vi "convert to deltaF-F.vi"(8 "error in (no error)":errorcluster, 11 "DAQOrcaFlash in":refnum<class "DAQOrcaFlash.lvclass">) -> (0 "error out":errorcluster, 3 "DAQOrcaFlash out":refnum<class "DAQOrcaFlash.lvclass">)   [LabVIEW 2012, in "DAQOrcaFlash.lvclass"]
uses:
  DAQOrcaFlash.lvclass
  dependencies/LabTIFF/LabTIFF/Opening Purpose.ctl
  DAQOrcaFlash.lvclass/DAQOrcaFlash.ctl
panel:
  out "min value":u32
  out "max value":u32
  out "file progress":dbl(slide) scale=0.0..1.0
  out "folder progress":dbl(slide) scale=0.0..1.0
  in  "cxd folder Path":path
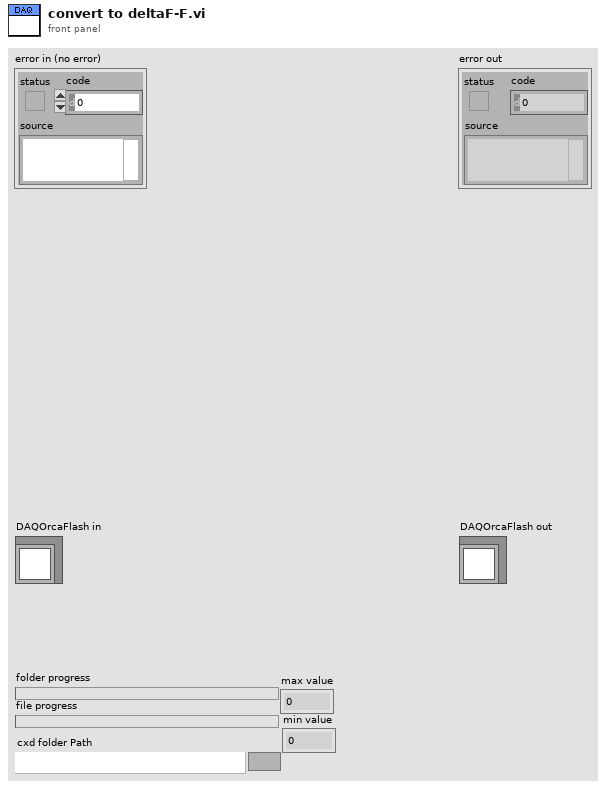
[diagram p1: front panel]
types:
  T1 = typedef "Opening Purpose.ctl" = enum16{"Read", "Write"}
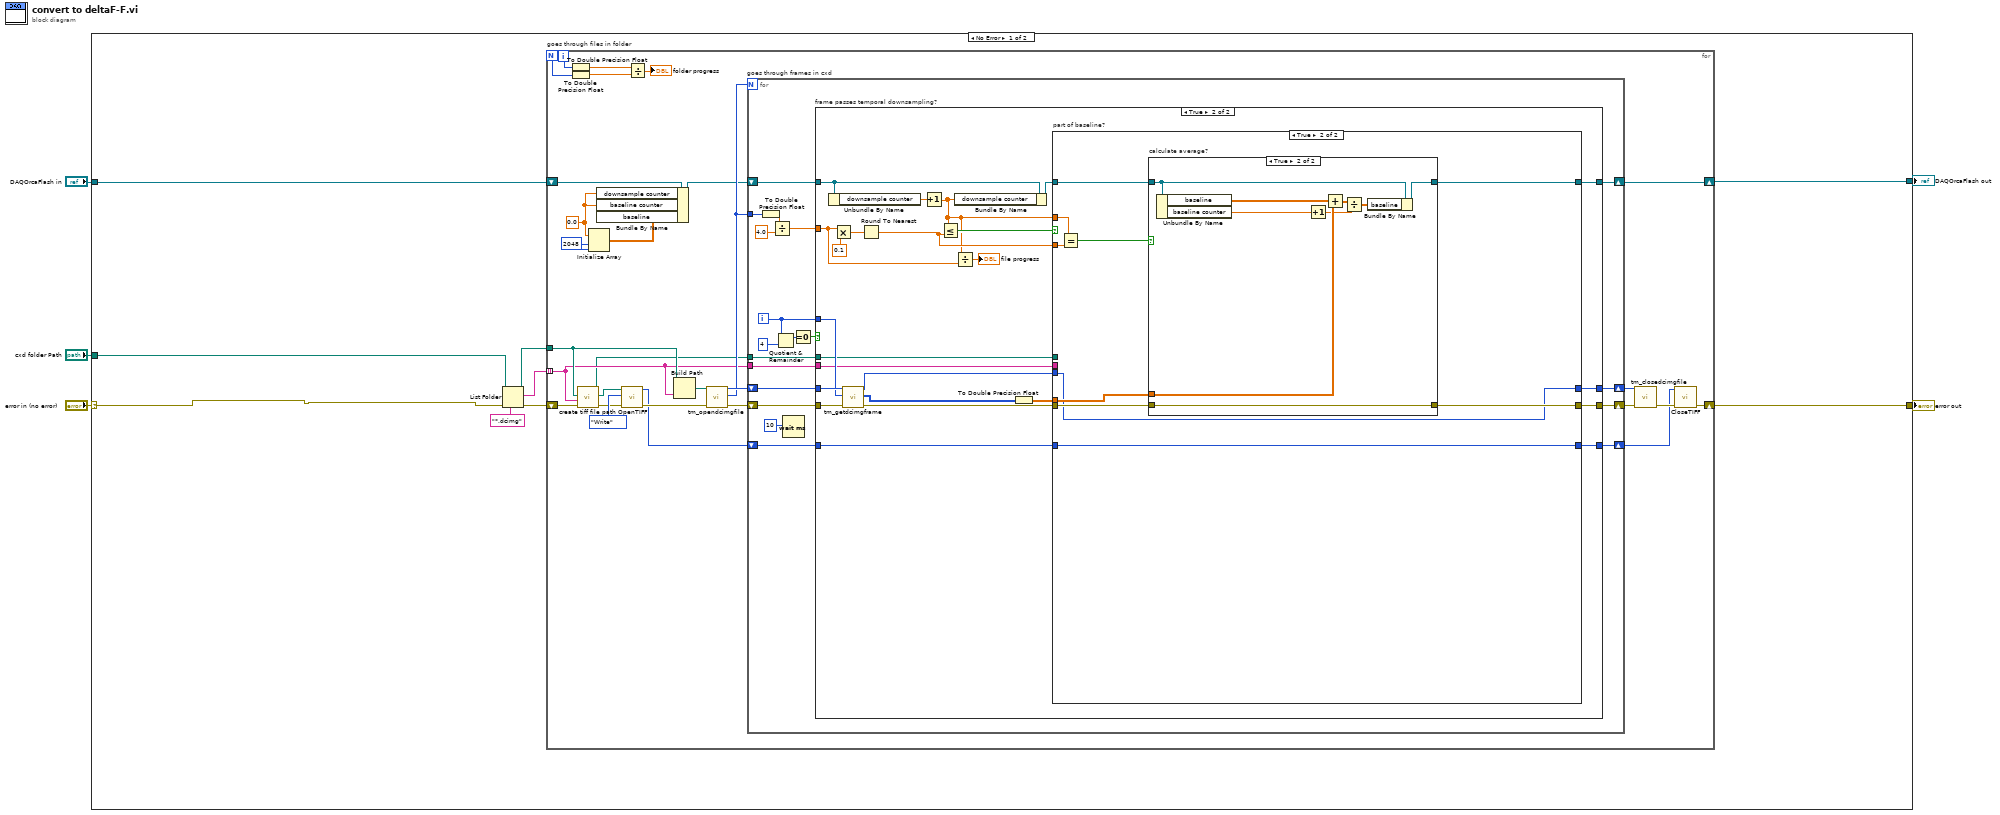
[diagram p0: block diagram]
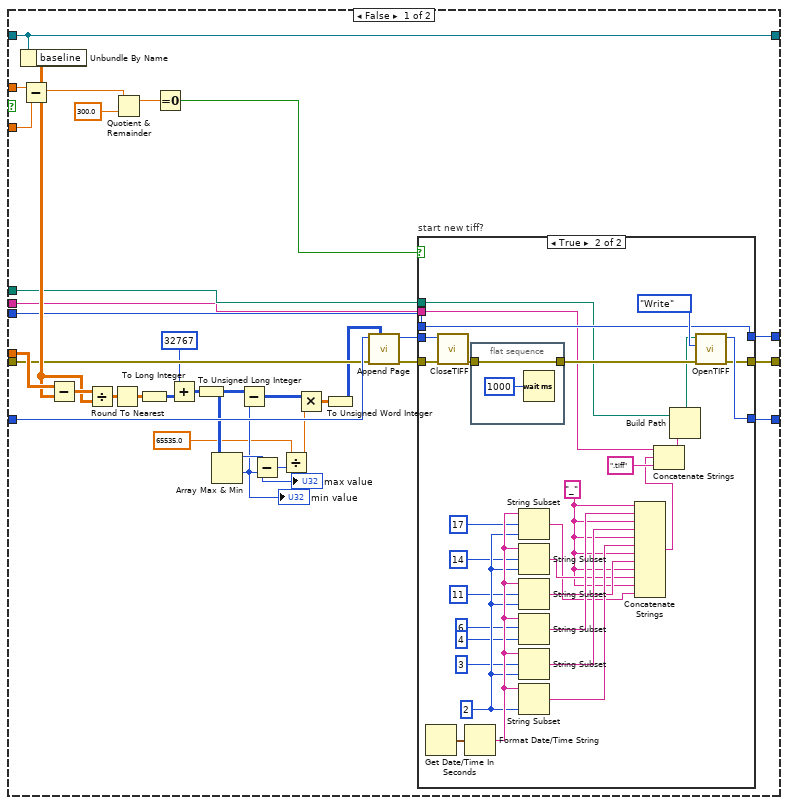
[diagram p3: hidden frame]
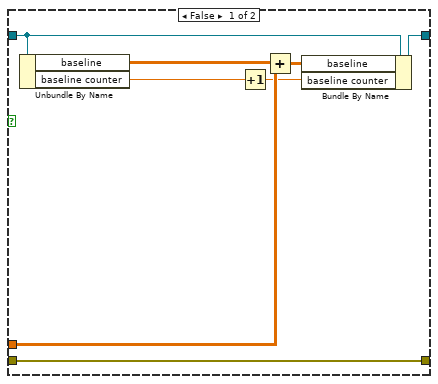
[diagram p5: hidden frame]
diagram:
  n1 = case shown="No Error" "error in (no error)" {
    selector: "error in (no error)" -> [w7 w188]
    tunnel: [w6 w188] -> w4
    tunnel: [w9 w187] -> w2
    tunnel: "DAQOrcaFlash in" -> [w10 w187]
    tunnel: "cxd folder Path" -> [w14 _]
    frame No Error {
      n2 = List Folder(path=w14, pattern="*.dcimg", error in=w7) -> (path out=w11:path, filenames=w12:string[], error out=w8:errorcluster)  [unwired: 1 in, 1 out]
      n3 = for "goes through files in folder" {
        N -> [w27]
        tunnel: w12 -> [w21] mode=indexing
        tunnel: w11 -> [w22]
        shift-right: [w39] -> w9
        shift-left: w10 -> [w38]
        shift-right: [w18] -> w6
        shift-left: w8 -> [w26]
        i -> [w29]
        w35 = 2048 ("dimension size")
        w34 = sgl 0.0 ("element")
        n4 = To Double Precision Float(number=w29) -> (double precision float=w30:dbl)
        n5 = To Double Precision Float(number=w27) -> (double precision float=w31:dbl)
        n6 = call "create tiff file path.vi"("error in (no error)"=w26, "dcimg name"=w21, "cxd folder Path"=w22) -> ("error IO"=w25:errorcluster, "tiff file path"=w24:path, "tiff folder path"=w15:path)  [unwired: 6 in]
        n7 = Initialize Array(w34, w35, w35) -> (w36:sgl[][])
        n8 = Bundle By Name(cluster=w38, "downsample counter"=w34, "baseline counter"=w34, "baseline"=w36) -> (w37:refnum<class "DAQOrcaFlash.lvclass">)
        n9 = call "OpenTIFF.vi"("error in (no error)"=w25, "Opening Purpose"=Opening_Purpose."Write", "File Path"=w24) -> ("error out"=w33:errorcluster, "TIFF File Ref"=w23:i32)  [unwired: 7 in]
        n10 = Divide(x=w30, y=w31) -> (x/y=→"folder progress":dbl)
        n11 = Build Path(base path=w22, name or relative path=w21) -> (appended path=w43:path)
        n12 = call <userlib>:"tm_opendcimgfile.vi"("error in (no error)"=w33, "Path"=w43) -> ("error out"=w42:errorcluster, "Total Frames"=w40:i32, "File Handle"=w41:u32)  [unwired: 7 in]
        n13 = for "goes through frames in cxd" {
          N: w40 -> [_]
          shift-right: [w44] -> w17
          shift-left: w41 -> [w58]
          shift-right: [w49] -> w19
          shift-left: w42 -> [w60]
          tunnel: w40 -> [w53]
          shift-right: [w55] -> w39
          shift-left: w37 -> [w56]
          shift-right: [w45] -> w16
          shift-left: w23 -> [w48]
          tunnel: w15 -> [w47]
          tunnel: w21 -> [w46]
          i -> [w57]
          n14 = To Double Precision Float(number=w53) -> (double precision float=w51:dbl)
          n15 = Divide(x=w51, y=4.0) -> (x/y=w50:dbl)
          n16 = Quotient & Remainder(x=w57, y=4) -> (x-y*floor(x/y)=w61:i32)  [unwired: 1 out]
          n17 = Wait (ms)(milliseconds to wait=u32 10 ("millisecond timer value")) -> ()  [unwired: 1 out]
          n18 = Equal To 0?(x=w61) -> (x = 0?=w59:bool)
          n19 = case "frame passes temporal downsampling?" shown="True" w59 {
            tunnel: w60 -> [w64 w90]
            tunnel: w58 -> [w63 w89]
            tunnel: w57 -> [_ w88]
            tunnel: w50 -> [_ w71]
            tunnel: w56 -> [w66 w85]
            tunnel: [w66 w86] -> w55
            tunnel: [w64 w82] -> w49
            tunnel: w48 -> [w65 w81]
            tunnel: w47 -> [_ w80]
            tunnel: w46 -> [_ w79]
            tunnel: [w65 w78] -> w45
            tunnel: [w63 w76] -> w44
            frame False {
            }
            frame True {
              n20 = Unbundle By Name(w85) -> ("downsample counter"=w83:dbl)
              n21 = Multiply(x=w71, y=0.1) -> (x*y=w74:dbl)
              n22 = call <userlib>:"tm_getdcimgframe.vi"("error in (no error)"=w90, "Frame Index"=w88, "File Handle in"=w89) -> ("error out"=w68:errorcluster, "Data"=w67:u16[][], "File Handle out"=w77:u32)  [unwired: 5 in, 1 out]
              n23 = Round To Nearest(number=w74) -> (nearest integer value=w73:dbl)
              n24 = Increment(x=w83) -> (x+1=w70:dbl)
              n25 = Less Or Equal?(x=w70, y=w73) -> (x <= y?=w87:bool)
              n26 = Bundle By Name(cluster=w85, "downsample counter"=w70) -> (w84:refnum<class "DAQOrcaFlash.lvclass">)
              n27 = Divide(x=w70, y=w71) -> (x/y=→"file progress":dbl)
              n28 = To Double Precision Float(number=w67) -> (double precision float=w69:dbl[][])
              n29 = case "part of baseline?" shown="True" w87 {
                tunnel: w68 -> [w103 w163]
                tunnel: w69 -> [w124 w169]
                tunnel: w84 -> [w106 w168]
                tunnel: [w106 w167] -> w86
                tunnel: w70 -> [w120 w166]
                tunnel: w73 -> [w119 w165]
                tunnel: [w110 w162] -> w82
                tunnel: w81 -> [w121 w161]
                tunnel: w80 -> [w113 _]
                tunnel: w79 -> [w112 _]
                tunnel: [w111 w161] -> w78
                tunnel: w77 -> [w109 w160]
                tunnel: [w108 w160] -> w76
                frame False {
                  n30 = Unbundle By Name(w106) -> ("baseline"=w122:dbl[][])
                  n31 = Subtract(x=w120, y=w119) -> (x-y=w107:dbl)
                  n32 = Subtract(x=w124, y=w122) -> (x-y=w123:dbl[][])
                  n33 = Divide(x=w123, y=w122) -> (x/y=w105:dbl[][])
                  n34 = Round To Nearest(number=w105) -> (nearest integer value=w104:dbl[][])
                  n35 = Quotient & Remainder(x=w107, y=300.0) -> (x-y*floor(x/y)=w118:dbl)  [unwired: 1 out]
                  n36 = To Long Integer(number=w104) -> (32bit integer=w102:i32[][])
                  n37 = Equal To 0?(x=w118) -> (x = 0?=w116:bool)
                  n38 = Add(x=32767, y=w102) -> (x+y=w100:i32[][])
                  n39 = To Unsigned Long Integer(number=w100) -> (unsigned 32bit integer=w99:u32[][])
                  n40 = Array Max & Min(array=w99) -> (max value=w98:u32, min value=w97:u32)  [unwired: 2 out]
                  "max value" <- w98
                  "min value" <- w97
                  n41 = Subtract(x=w99, y=w97) -> (x-y=w94:u32[][])
                  n42 = Subtract(x=w98, y=w97) -> (x-y=w95:u32)
                  n43 = Divide(x=65535.0, y=w95) -> (x/y=w93:dbl)
                  n44 = Multiply(x=w94, y=w93) -> (x*y=w92:dbl[][])
                  n45 = To Unsigned Word Integer(number=w92) -> (unsigned 16bit integer=w91:u16[][])
                  n46 = call "Append Page.vi"("U16 Image"=w91, "error in (no error)"=w103, "TIFF File Ref"=w121) -> ("error out"=w115:errorcluster, "TIFF File Ref out"=w114:i32)  [unwired: 7 in]
                  n47 = case "start new tiff?" shown="True" w116 {
                    tunnel: w115 -> [w126 w157]
                    tunnel: w114 -> [w127 w156]
                    tunnel: w113 -> [_ w128]
                    tunnel: w112 -> [_ w129]
                    tunnel: [w127 w153] -> w111
                    tunnel: [w126 w152] -> w110
                    tunnel: w109 -> [w125 w151]
                    tunnel: [w125 w151] -> w108
                    frame False {
                    }
                    frame True {
                      w131 = "_" ("string")
                      w145 = 2 ("length (rest)")
                      n48 = Get Date/Time In Seconds() -> (seconds since 1Jan1904=w149:timestamp)
                      n49 = call "CloseTIFF.vi"("error in (no error)"=w157, "TIFF File Ref"=w156) -> ("error out"=w155:errorcluster)  [unwired: 9 in]
                      n50 = Format Date/Time String(seconds (now)=w149) -> (date/time string=w146:string)  [unwired: 2 in]
                      n51 = flat-sequence {
                        tunnel: w155 -> [w158]
                        tunnel: [w158] -> w150
                        frame #0 {
                          n52 = Wait (ms)(milliseconds to wait=u32 1000) -> ()  [unwired: 1 out]
                        }
                      }
                      n53 = String Subset(string=w146, offset (0)=17, length (rest)=w145) -> (substring=w133:string)
                      n54 = String Subset(string=w146, offset (0)=14, length (rest)=w145) -> (substring=w134:string)
                      n55 = String Subset(string=w146, offset (0)=11, length (rest)=w145) -> (substring=w135:string)
                      n56 = String Subset(string=w146, offset (0)=6, length (rest)=4 ("length (rest)")) -> (substring=w138:string)
                      n57 = String Subset(string=w146, offset (0)=3, length (rest)=w145) -> (substring=w137:string)
                      n58 = String Subset(string=w146, length (rest)=w145) -> (substring=w136:string)  [unwired: 1 in]
                      n59 = Concatenate Strings(w131, w138, w131, w137, w131, w136, w131, w135, w131, w134, w131, w133) -> (w132:string)
                      n60 = Concatenate Strings(w129, w132, ".tiff" ("search string/char (-)")) -> (w147:string)
                      n61 = Build Path(base path=w128, name or relative path=w147) -> (appended path=w130:path)
                      n62 = call "OpenTIFF.vi"("error in (no error)"=w150, "Opening Purpose"=Opening_Purpose."Write", "File Path"=w130) -> ("error out"=w152:errorcluster, "TIFF File Ref"=w153:i32)  [unwired: 7 in]
                    }
                  }
                }
                frame True {
                  n63 = Equal?(x=w166, y=w165) -> (x = y?=w164:bool)
                  n64 = case "calculate average?" shown="True" w164 {
                    tunnel: w169 -> [w176 w185]
                    tunnel: w168 -> [w174 w183]
                    tunnel: [w173 w182] -> w167
                    tunnel: w163 -> [w170 w181]
                    tunnel: [w170 w181] -> w162
                    frame False {
                      n65 = Unbundle By Name(w174) -> ("baseline"=w177:dbl[][], "baseline counter"=w175:dbl)
                      n66 = Increment(x=w175) -> (x+1=w171:dbl)
                      n67 = Add(x=w177, y=w176) -> (x+y=w172:dbl[][])
                      n68 = Bundle By Name(cluster=w174, "baseline"=w172, "baseline counter"=w171) -> (w173:refnum<class "DAQOrcaFlash.lvclass">)
                    }
                    frame True {
                      n69 = Unbundle By Name(w183) -> ("baseline"=w186:dbl[][], "baseline counter"=w184:dbl)
                      n70 = Increment(x=w184) -> (x+1=w180:dbl)
                      n71 = Add(x=w186, y=w185) -> (x+y=w179:dbl[][])
                      n72 = Divide(x=w179, y=w180) -> (x/y=w178:dbl[][])
                      n73 = Bundle By Name(cluster=w183, "baseline"=w178) -> (w182:refnum<class "DAQOrcaFlash.lvclass">)
                    }
                  }
                }
              }
            }
          }
        }
        n74 = call <userlib>:"tm_closedcimgfile.vi"("error in (no error)"=w19, "File Handle"=w17) -> ("error out"=w20:errorcluster)  [unwired: 9 in]
        n75 = call "CloseTIFF.vi"("error in (no error)"=w20, "TIFF File Ref"=w16) -> ("error out"=w18:errorcluster)  [unwired: 9 in]
      }
    }
    frame Error {
    }
  }
  "error out" <- w4
  "DAQOrcaFlash out" <- w2
